vi "Restart Application.vi"(8 "error in (no error)":errorcluster) -> (0 "error out":errorcluster)   [LabVIEW 2016, in "SLL Application.lvlib"]
doc: "Shuts down and restarts the current application."
uses:
  SLL Application.lvlib
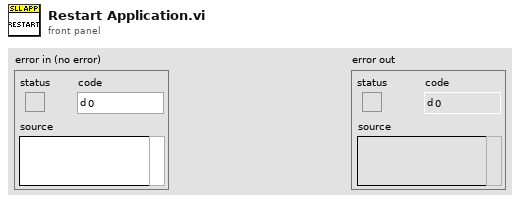
[diagram p1: front panel]
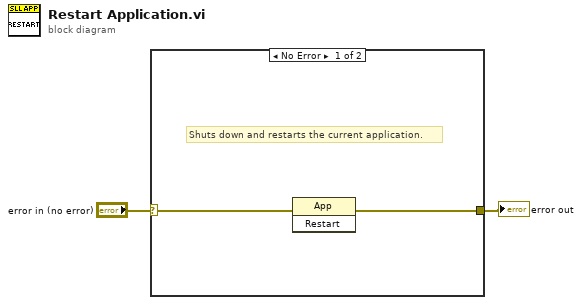
[diagram p0: block diagram]
diagram:
  n1 = case shown="No Error" "error in (no error)" {
    selector: "error in (no error)" -> [w4 w5]
    tunnel: [w3 w5] -> w1
    frame No Error {
      # "Shuts down and restarts the current application."
      n2 = invoke class="App" method="Restart"(error in=w4) -> (error out=w3:errorcluster)  [unwired: 2 in, 2 out]
    }
    frame Error {
    }
  }
  "error out" <- w1
